vi "global_log_file.vi"() -> ()   [LabVIEW 2013]
panel:
  out "Log File (global)":string
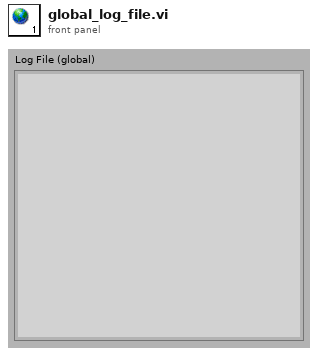
[diagram p1: front panel]
diagram:
